vi "HandleDeadband.vi"(7 "Deadband":dbl, 11 "Input":dbl) -> (3 "Output":dbl)   [LabVIEW 2020]
doc: "If the input is within the deadband, outputs 0. Otherwise outputs the input"
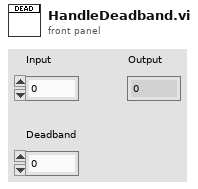
[diagram p1: front panel]
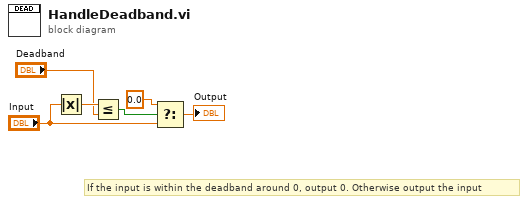
[diagram p0: block diagram]
diagram:
  # "If the input is within the deadband around 0, output 0. Otherwise output the input"
  n1 = Absolute Value(x="Input") -> (abs(x)=w6:dbl)
  n2 = Less Or Equal?(x=w6, y="Deadband") -> (x <= y?=w4:bool)
  n3 = Select(t=0.0, s=w4, f="Input") -> (s? t:f=→"Output":dbl)
